vi "Extract Control Text.vi"(8 "error in (no error)":errorcluster, 9 "Label Prefix":string, 10 "ControlRefs[]":refnum<vi>[](array[refnum]), 11 "VI Data in":refnum<class "VI Data.lvclass">) -> (0 "error out":errorcluster, 3 "VI Data out":refnum<class "VI Data.lvclass">)   [LabVIEW 2013, in "SET Project Data.lvlib" / "VI Data.lvclass"]
uses:
  VI Data.lvclass
  VI Data.lvclass/VI Data.ctl
  Control Classes/GObject/GObject.lvclass
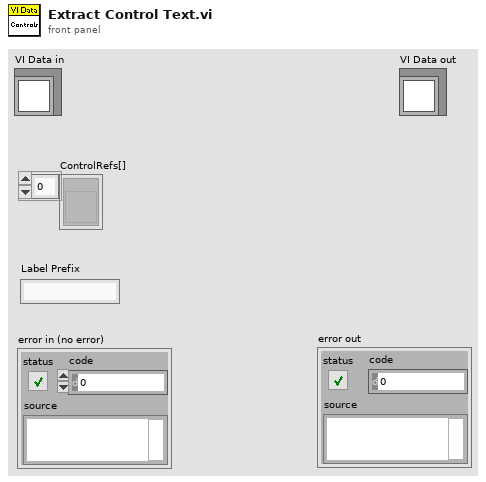
[diagram p1: front panel]
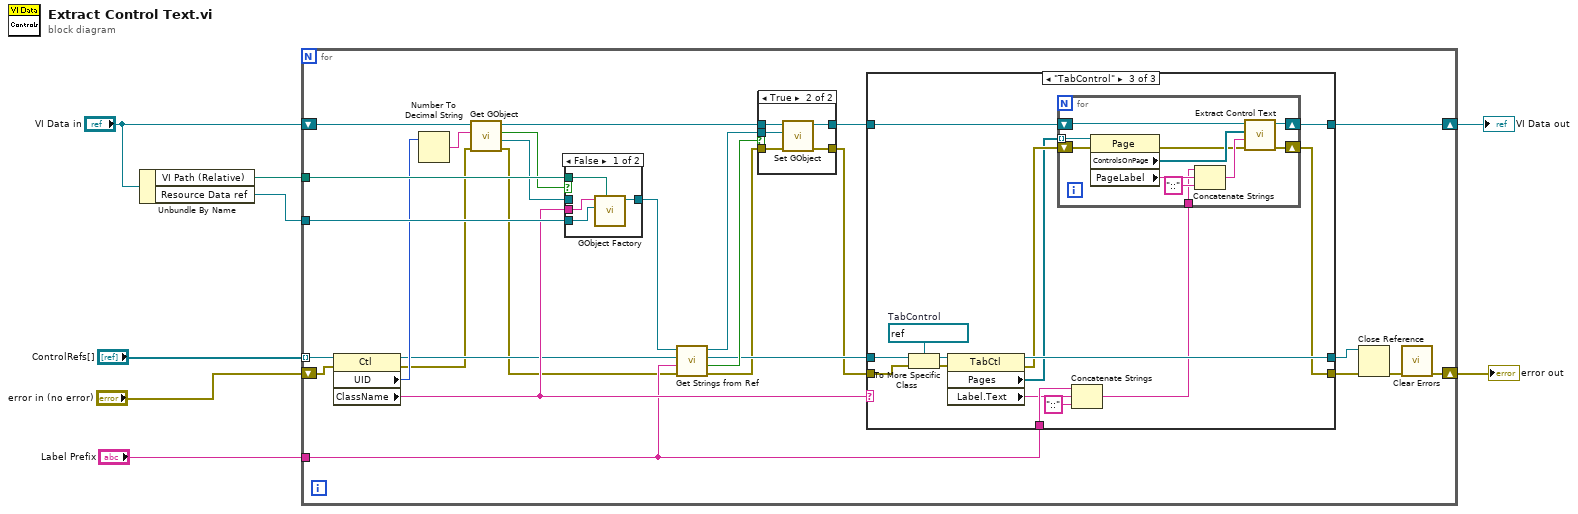
[diagram p0: block diagram]
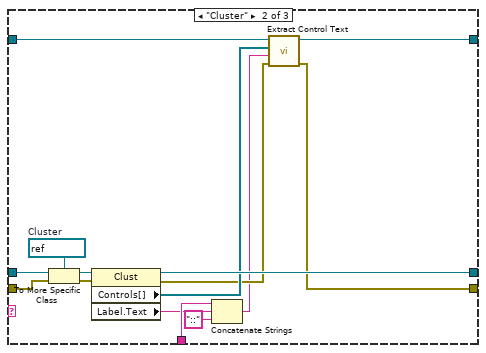
[diagram p5: hidden frame]
diagram:
  n1 = Unbundle By Name("VI Data in") -> ("VI Path (Relative)"=w4:path, "Resource Data ref"=w3:refnum<data-value>)
  n2 = for {
    tunnel: "ControlRefs[]" -> [w31] mode=indexing
    shift-right: [w35] -> w6
    shift-left: "error in (no error)" -> [w30]
    tunnel: "Label Prefix" -> [w25]
    tunnel: w3 -> [w34]
    tunnel: w4 -> [w32]
    shift-right: [w10] -> w2
    shift-left: "VI Data in" -> [w9]
    n3 = property class="Ctl"(reference=w31, error in=w30) -> (reference out=w26:refnum<vi>, error out=w17:errorcluster, "UID"=w28:i32, "ClassName"=w29:string)
    n4 = Number To Decimal String(number=w28) -> (decimal integer string=w23:string)  [unwired: 1 in]
    n5 = call-dynamic "Get GObject.vi"("error in (no error)"=w17, "GObject UID"=w23, "VI Data in"=w9) -> ("error out"=w16:errorcluster, "GObject"=w21:refnum<class "GObject.lvclass">, "found"=w22:bool, "VI Data out"=w20:refnum<class "VI Data.lvclass">)  [unwired: 5 in]
    n6 = case shown="False" w22 {
      tunnel: [w46 w47] -> w27
      tunnel: w34 -> [w44 _]
      tunnel: w32 -> [w43 _]
      tunnel: w29 -> [w45 _]
      tunnel: w21 -> [_ w47]
      frame False {
        n7 = call "GObject Factory.vi"("Owning VI"=w43, "LangFile ref"=w44, "ClassName"=w45) -> ("GObject"=w46:refnum<class "GObject.lvclass">)  [unwired: 8 in]
      }
      frame True {
      }
    }
    n8 = call-dynamic "Get Strings from Ref.vi"("error in (no error)"=w16, "Label Prefix"=w25, "GObj Refnum in"=w26, "GObject in"=w27) -> ("error out"=w13:errorcluster, "Valid?"=w15:bool, "GObj Refnum out"=w14:refnum<vi>, "GObject out"=w18:refnum<class "GObject.lvclass">)  [unwired: 3 in, 1 out]
    n9 = case shown="True" w15 {
      tunnel: w20 -> [w36 w42]
      tunnel: w18 -> [_ w41]
      tunnel: w13 -> [w37 w40]
      tunnel: [w37 w39] -> w12
      tunnel: [w36 w38] -> w19
      frame False {
      }
      frame True {
        n10 = call "Set GObject.vi"("error in (no error)"=w40, "GObject.lvclass"=w41, "VI Data in"=w42) -> ("error out"=w39:errorcluster, "VI Data out"=w38:refnum<class "VI Data.lvclass">)  [unwired: 6 in, 1 out]
      }
    }
    n11 = case shown="\"TabControl\"" w29 {
      tunnel: w14 -> [w50 w65 w80]
      tunnel: [w50 w60 w75] -> w24
      tunnel: [w48 w59 w74] -> w10
      tunnel: w12 -> [w49 w64 w79]
      tunnel: [w49 w56 w72] -> w11
      tunnel: w25 -> [_ w53 w69]
      tunnel: w19 -> [w48 w51 w66]
      frame "Control", Default {
      }
      frame "Cluster" {
        w63 = refnum<vi> refnum  # Cluster
        n12 = To More Specific Class(target class=w63, reference=w65, error in=w64) -> (specific class reference=w62:refnum<vi>, error out=w61:errorcluster)
        n13 = property class="Clust"(reference=w62, error in=w61) -> (reference out=w60:refnum<vi>, error out=w57:errorcluster, "Controls[]"=w58:refnum<vi>[], "Label.Text"=w52:string)
        n14 = Concatenate Strings(w53, w52, "::" ("string")) -> (w54:string)
        n15 = call "Extract Control Text.vi"("error in (no error)"=w57, "Label Prefix"=w54, "ControlRefs[]"=w58, "VI Data in"=w51) -> ("error out"=w56:errorcluster, "VI Data out"=w59:refnum<class "VI Data.lvclass">)  [unwired: 6 in]
      }
      frame "TabControl" {
        w78 = refnum<vi> refnum  # TabControl
        n16 = To More Specific Class(target class=w78, reference=w80, error in=w79) -> (specific class reference=w77:refnum<vi>, error out=w76:errorcluster)
        n17 = property class="TabCtl"(reference=w77, error in=w76) -> (reference out=w75:refnum<vi>, error out=w73:errorcluster, "Pages"=w67:refnum<vi>[], "Label.Text"=w68:string)
        n18 = Concatenate Strings(w69, w68, "::" ("string")) -> (w70:string)
        n19 = for {
          tunnel: w70 -> [w83]
          shift-right: [w90] -> w74
          shift-left: w66 -> [w91]
          shift-right: [w89] -> w72
          shift-left: w73 -> [w86]
          tunnel: w67 -> [w87] mode=indexing
          n20 = property class="Page"(reference=w87, error in=w86) -> (error out=w81:errorcluster, "ControlsOnPage"=w88:refnum<vi>[], "PageLabel"=w85:string)  [unwired: 1 out]
          n21 = Concatenate Strings(w83, w85, "::" ("string")) -> (w82:string)
          n22 = call "Extract Control Text.vi"("error in (no error)"=w81, "Label Prefix"=w82, "ControlRefs[]"=w88, "VI Data in"=w91) -> ("error out"=w89:errorcluster, "VI Data out"=w90:refnum<class "VI Data.lvclass">)  [unwired: 6 in]
        }
      }
    }
    n23 = Close Reference(reference=w24, error in (no error)=w11) -> (error out=w33:errorcluster)
    n24 = call <vilib>:"Clear Errors.vi"("error in (no error)"=w33) -> ("error out"=w35:errorcluster)  [unwired: 6 in]
  }
  "error out" <- w6
  "VI Data out" <- w2
